vi "GetTableSelect.vi"(6 "キー列(0)":i32, 8 "error in (no error)":errorcluster caption="エラー入力（エラーなし）", 11 "Table ref":refnum<vi>) -> (0 "error out":errorcluster caption="エラー出力", 1 "選択行[]":i32[](array[numeric]), 2 "選択文字[]":string[](array[string]), 3 "Table ref (copy)":refnum<vi>, 4 "選択行有り?":bool)   [LabVIEW 2014]
uses:
  <vilib>/Utility/miscctls.llb/LVRowAndColumnTypeDef.ctl
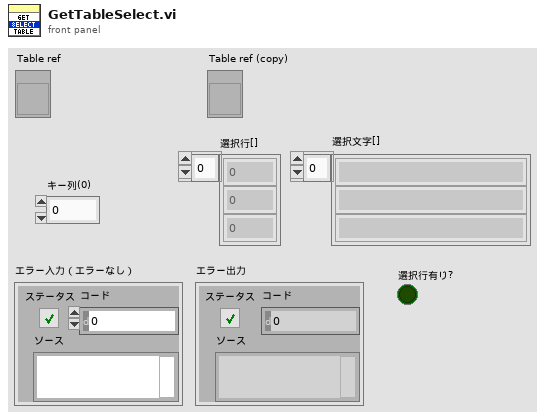
[diagram p1: front panel]
types:
  T1 = typedef "LVRowAndColumnTypeDef.ctl" = cluster{"Row":i32, "Column":i32}
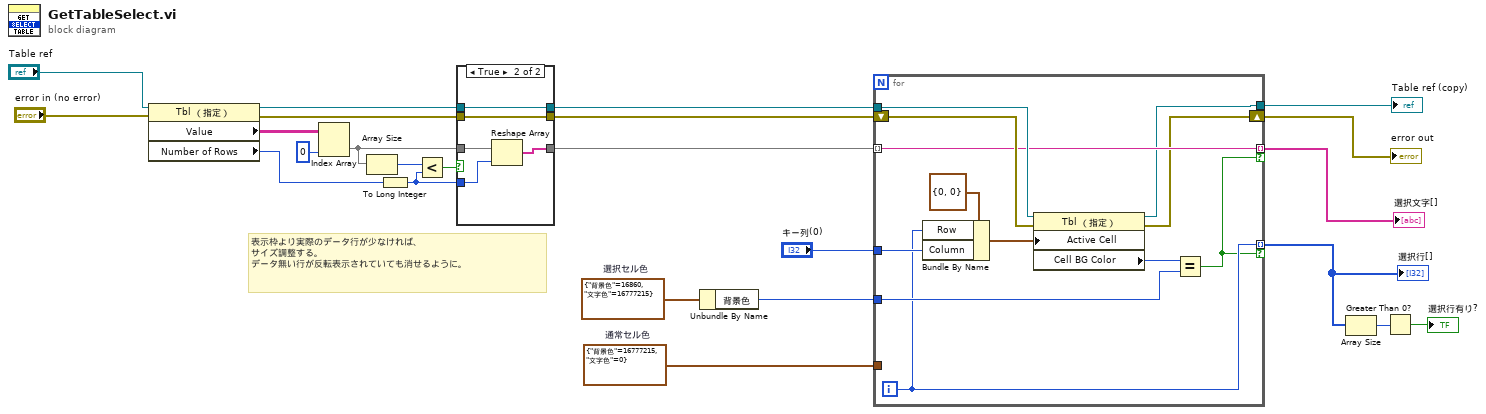
[diagram p0: block diagram]
diagram:
  w7 = cluster{"背景色":u32, "文字色":u32} {"背景色"=16860, "文字色"=16777215}  # 選択セル色
  w5 = cluster{"背景色":u32, "文字色":u32} {"背景色"=16777215, "文字色"=0}  # 通常セル色
  # "表示枠より実際のデータ行が少なければ、\nサイズ調整する。\nデータ無い行が反転表示されていても消せるように。"
  n1 = property class="Tbl （指定）"(reference="Table ref", error in="error in (no error)") -> (reference out=w10:refnum<vi>, error out=w12:errorcluster, "Value"=w24:string[][], "Number of Rows"=w16:u32)
  n2 = Index Array(array=w24, index (col)=0 ("無効な指標 （列）")) -> (element=w18:string[])  [unwired: 1 in]
  n3 = Array Size(array=w18) -> (size(s)=w17:i32)
  n4 = To Long Integer(number=w16) -> (32bit integer=w15:i32)
  n5 = Less?(x=w17, y=w15) -> (x < y?=w14:bool)
  n6 = case shown="TRUE" w14 {
    tunnel: [w25 w32] -> w9
    tunnel: w18 -> [w25 w31]
    tunnel: w15 -> [_ w30]
    tunnel: [w26 w29] -> w13
    tunnel: w12 -> [w26 w29]
    tunnel: [w27 w28] -> w11
    tunnel: w10 -> [w27 w28]
    frame False {
    }
    frame True {
      n7 = Reshape Array(w31, w30) -> (w32:string[])
    }
  }
  n8 = Unbundle By Name(w7) -> ("背景色"=w6:u32)
  n9 = for {
    tunnel: w11 -> [w41]
    shift-right: [w34] -> w21
    shift-left: w13 -> [w40]
    tunnel: [w33] -> w20
    tunnel: w9 -> [w37] mode=indexing
    tunnel: "キー列(0)" -> [w43]
    tunnel: w6 -> [w38]
    tunnel: w5 -> [_]
    tunnel: [w37] -> w4 mode=indexing if=w35
    tunnel: [w36] -> w3 mode=indexing if=w35
    i -> [w36]
    n10 = Bundle By Name(cluster=T1 {"Row"=0, "Column"=0} ("行列指定"), "Row"=w36, "Column"=w43) -> (w42:T1)
    n11 = property class="Tbl （指定）"(reference=w41, error in=w40, "Active Cell"=w42) -> (reference out=w33:refnum<vi>, error out=w34:errorcluster, "Cell BG Color"=w39:u32)
    n12 = Equal?(x=w39, y=w38) -> (x = y?=w35:bool)
  }
  "error out" <- w21
  "Table ref (copy)" <- w20
  "選択文字[]" <- w4
  "選択行[]" <- w3
  n13 = Array Size(array=w3) -> (size(s)=w2:i32)
  n14 = Greater Than 0?(x=w2) -> (x > 0?=→"選択行有り?":bool)
